vi "query.vi"(2 "Condition":string, 3 "errorIn":errorcluster, 4 "Table Name":string, 5 "Connection Name":string) -> (0 "errorOut":errorcluster, 1 "data":string[][](array[string]))   [LabVIEW 2020, in "databaseLibrary.lvlib"]
uses:
  databaseLibrary.lvlib
  <vilib>/addons/database/Connection.llb/DB Tools Open Connec (String).vi
  <vilib>/addons/database/_DB Variant To Data/Database Variant To Data.xnode
  <vilib>/addons/database/NI_Database_API.lvlib
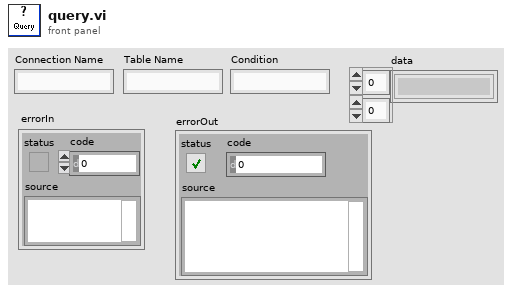
[diagram p1: front panel]
types:
  T1 = typedef "NI_Database_API.lvlib/Conn ObjectReference.ctl" = refnum<k1>
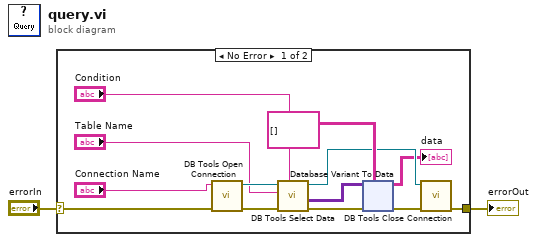
[diagram p0: block diagram]
diagram:
  n1 = case shown="No Error" "errorIn" {
    selector: "errorIn" -> [w3 w60]
    tunnel: [w10 w60] -> w2
    frame No Error {
      n2 = call-poly <vilib>:"DB Tools Open Connection.vi"("error in (no error)"=w3, "connection information"="Connection Name") -> ("error out"=w8:errorcluster, "connection reference"=w7:T1)  [unwired: 6 in]
      n3 = call <vilib>:"DB Tools Select Data.vi"("condition"="Condition", "error in (no error)"=w8, "table"="Table Name", "connection reference"=w7) -> ("error out"=w14:errorcluster, "data"=w15:variant[][], "connection reference out"=w9:T1)  [unwired: 2 in]
      n4 = xnode "Database Variant To Data"("database variant"=w15, "error in (no error)"=w14, "type"=string[][] []) -> ("data"=→"data":string[][], "error out"=w11:errorcluster)
      n5 = call <vilib>:"DB Tools Close Connection.vi"("error in (no error)"=w11, "connection reference"=w9) -> ("error out"=w10:errorcluster)  [unwired: 5 in]
    }
    frame Error {
    }
  }
  "errorOut" <- w2
